vi "Configure.vi"(8 "error in (no error)":errorcluster, 10 "I2C User Configuration":T1, 11 "I2C Ref In":T3={"myRIO Reference"={"myRIO Model"=enum."Unknown", "myRIO Hardware Reference"={"Generic FPGA Reference"=refnum, "Allow multiple opens"=FALSE}}, "I2C Channels Enum"=enum."Not Connected", "I2C Configuration"={"I2C Transfer Rate"=enum."Fast mode (400 kbps)"}}) -> (0 "error out":errorcluster, 3 "I2C Ref Out":T3={"myRIO Reference"={"myRIO Model"=enum."Unknown", "myRIO Hardware Reference"={"Generic FPGA Reference"=refnum, "Allow multiple opens"=FALSE}}, "I2C Channels Enum"=enum."Not Connected", "I2C Configuration"={"I2C Transfer Rate"=enum."Fast mode (400 kbps)"}})   [LabVIEW 2021, in "I2C.lvlib"]
doc: "Configures the transfer rate of an Inter-Integrated Circuit (I2C) channel based on the input I2C reference."
uses:
  <vilib>/myRIO/Instrument Drivers/Onboard IO/I2C/I2C.lvlib
  <vilib>/myRIO/Instrument Drivers/Onboard IO/I2C/typedefs/I2C Reference.ctl
  <vilib>/myRIO/Common/Instrument Driver Framework/Utilities/typedefs/myRIO Generic Hardware Reference.ctl
  <vilib>/myRIO/Common/Instrument Driver Framework/Utilities/typedefs/Hardware Version Enum.ctl
  <vilib>/myRIO/Common/Instrument Driver Framework/Utilities/typedefs/myRIO v1.0 Reference.ctl
  <vilib>/myRIO/Common/Instrument Driver Framework/Utilities/typedefs/Generic FPGA Reference.ctl
  <vilib>/myRIO/Common/Instrument Driver Framework/myRIO v1.0/I2C/typedefs/I2C Channels Enum.ctl
  <vilib>/myRIO/Instrument Drivers/Onboard IO/I2C/typedefs/I2C Configuration.ctl
  <vilib>/myRIO/Instrument Drivers/Onboard IO/I2C/typedefs/I2C Transfer Rate.ctl
  <vilib>/myRIO/Instrument Drivers/Onboard IO/I2C/typedefs/I2C User Configuration.ctl
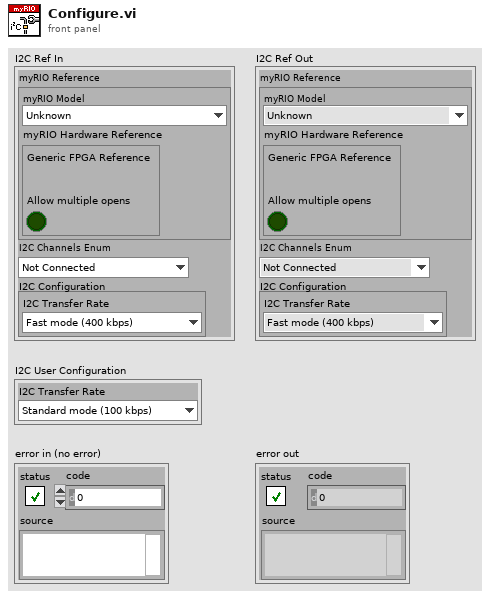
[diagram p1: front panel]
types:
  T1 = typedef "I2C.lvlib/I2C User Configuration.ctl" = cluster{"I2C Transfer Rate":T2}
  T2 = typedef "I2C.lvlib/I2C Transfer Rate.ctl" = enum16{"Standard mode (100 kbps)", "Fast mode (400 kbps)"}
  T3 = typedef "I2C.lvlib/I2C Reference.ctl" = cluster{"myRIO Reference":T4, "I2C Channels Enum":T8, "I2C Configuration":T9}
  T4 = typedef "myRIO Generic Hardware Reference.ctl" = cluster{"myRIO Model":T5, "myRIO Hardware Reference":T6}
  T5 = typedef "Hardware Version Enum.ctl" = enum16{"Unknown", "myRIO-1900", "myRIO-1950", "roboRIO", "NI ELVIS RIO CM", "ELVIS III"}
  T6 = typedef "myRIO v1.0 Reference.ctl" = cluster{"Generic FPGA Reference":T7, "Allow multiple opens":bool}
  T7 = typedef "Generic FPGA Reference.ctl" = refnum<k20>
  T8 = typedef "I2C Channels Enum.ctl" = enum16{"Not Connected", "A/I2C", "B/I2C", "I2C/I2C"}
  T9 = typedef "I2C.lvlib/I2C Configuration.ctl" = cluster{"I2C Transfer Rate":T2}
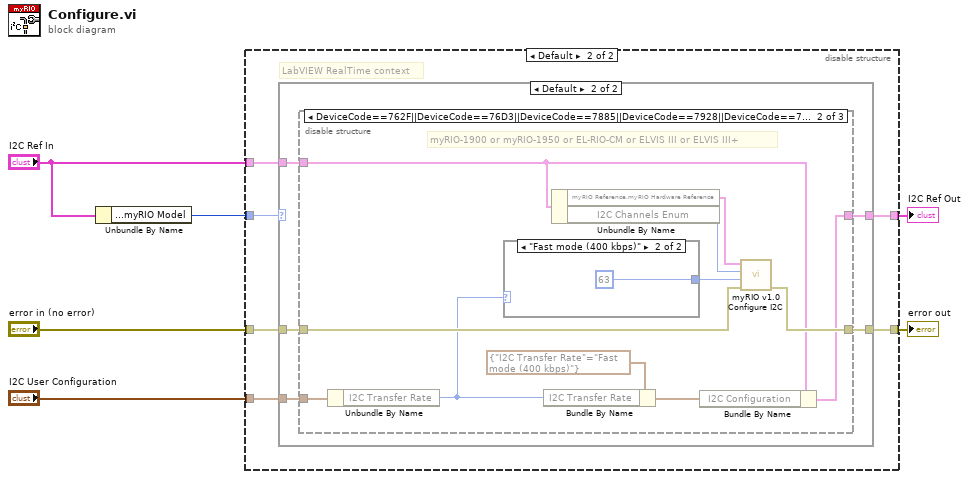
[diagram p0: block diagram]
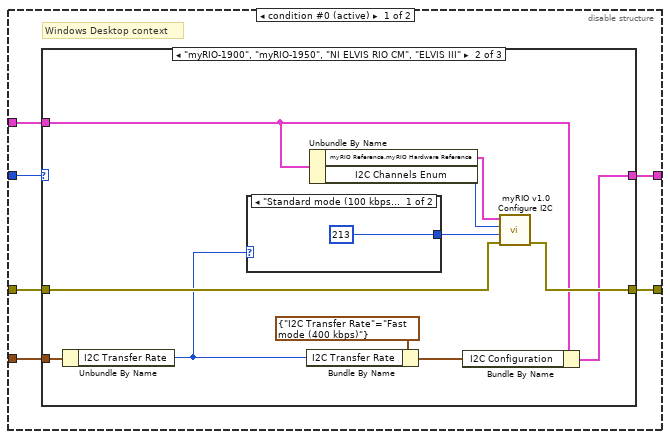
[diagram p2: hidden frame]
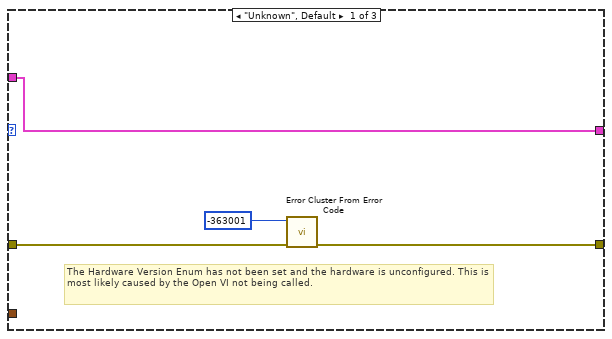
[diagram p3: hidden frame]
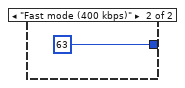
[diagram p4: hidden frame]
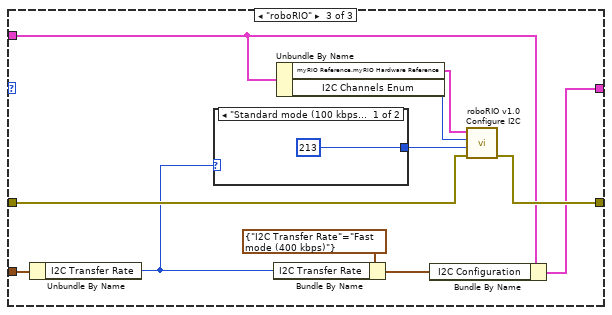
[diagram p5: hidden frame]
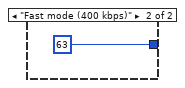
[diagram p6: hidden frame]
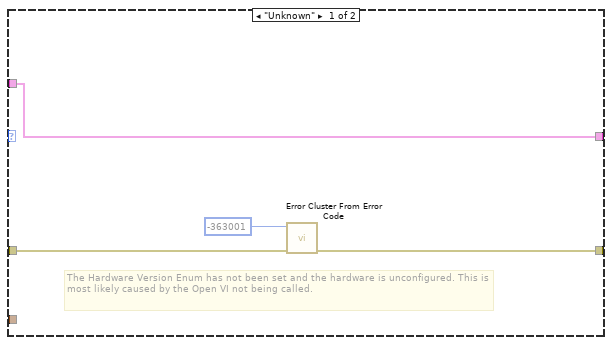
[diagram p7: hidden frame]
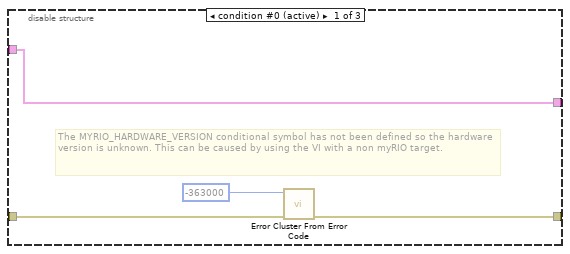
[diagram p8: hidden frame]
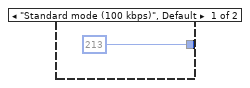
[diagram p9: hidden frame]
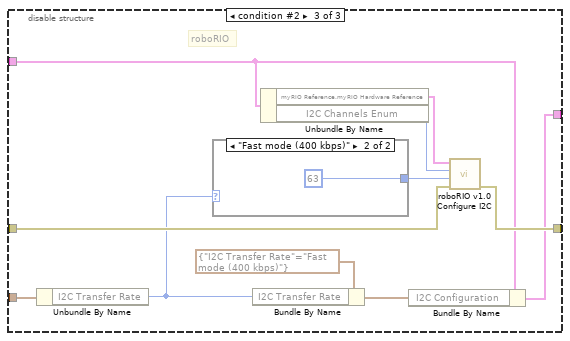
[diagram p10: hidden frame]
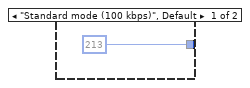
[diagram p11: hidden frame]
diagram:
  n1 = Unbundle By Name("I2C Ref In") -> ("myRIO Reference.myRIO Model"=w1:T5)
  n2 = disable-structure shown="Default" {
    disable-tunnel: [w12 w48] -> w6
    disable-tunnel: [w11 w47] -> w5
    disable-tunnel: "I2C User Configuration" -> [w10 w46]
    disable-tunnel: "I2C Ref In" -> [w9 w45]
    disable-tunnel: "error in (no error)" -> [w8 w44]
    disable-tunnel: w1 -> [w7 w43]
    frame condition #0 (active) {
      # "Windows Desktop context"
      n3 = case shown="\"myRIO-1900\", \"myRIO-1950\", \"NI ELVIS RIO CM\", \"ELVIS III\"" w7 {
        tunnel: [w15 w27 w40] -> w12
        tunnel: [w13 w26 w39] -> w11
        tunnel: w9 -> [w13 w21 w34]
        tunnel: w8 -> [w14 w25 w38]
        tunnel: w10 -> [_ w22 w35]
        frame "Unknown", Default {
          # "The Hardware Version Enum has not been set and the hardware is unconfigured. This is most likely caused by the Open VI not being called."
          n4 = call <vilib>:"Error Cluster From Error Code.vi"("error in (no error)"=w14, "error code (0)"=-363001) -> ("error out"=w15:errorcluster)  [unwired: 7 in]
        }
        frame "myRIO-1900", "myRIO-1950", "NI ELVIS RIO CM", "ELVIS III" {
          n5 = Unbundle By Name(w22) -> ("I2C Transfer Rate"=w18:T2)
          n6 = case shown="\"Standard mode (100 kbps)\", Default" w18 {
            tunnel: [u8 213 ("I2C Counter Value") u8 63 ("I2C Counter Value")] -> w17
            frame "Standard mode (100 kbps)", Default {
            }
            frame "Fast mode (400 kbps)" {
            }
          }
          n7 = Bundle By Name(cluster=T9 {"I2C Transfer Rate"=enum."Fast mode (400 kbps)"} ("I2C Configuration"), "I2C Transfer Rate"=w18) -> (w19:T9)
          n8 = Unbundle By Name(w21) -> ("myRIO Reference.myRIO Hardware Reference"=w23:T6, "I2C Channels Enum"=w24:T8)
          n9 = Bundle By Name(cluster=w21, "I2C Configuration"=w19) -> (w26:T3)
          n10 = call <vilib>:"myRIO v1.0 Configure I2C.vi"("error in (no error)"=w25, "I2C Counter Value"=w17, "Channel"=w24, "myRIO Ref In"=w23) -> ("error out"=w27:errorcluster)  [unwired: 6 in, 1 out]
        }
        frame "roboRIO" {
          n11 = Unbundle By Name(w35) -> ("I2C Transfer Rate"=w31:T2)
          n12 = case shown="\"Standard mode (100 kbps)\", Default" w31 {
            tunnel: [u8 213 ("I2C Counter Value") u8 63 ("I2C Counter Value")] -> w30
            frame "Standard mode (100 kbps)", Default {
            }
            frame "Fast mode (400 kbps)" {
            }
          }
          n13 = Bundle By Name(cluster=T9 {"I2C Transfer Rate"=enum."Fast mode (400 kbps)"} ("I2C Configuration"), "I2C Transfer Rate"=w31) -> (w32:T9)
          n14 = Unbundle By Name(w34) -> ("myRIO Reference.myRIO Hardware Reference"=w36:T6, "I2C Channels Enum"=w37:T8)
          n15 = Bundle By Name(cluster=w34, "I2C Configuration"=w32) -> (w39:T3)
          n16 = call <vilib>:"roboRIO v1.0 Configure I2C.vi"("error in (no error)"=w38, "I2C Counter Value"=w30, "Channel"=w37, "myRIO Ref In"=w36) -> ("error out"=w40:errorcluster)  [unwired: 6 in, 1 out]
        }
      }
    }
    frame condition #1 {
      # "LabVIEW RealTime context"
      n17 = case shown="Default" w43 {
        tunnel: [w51 w57] -> w48
        tunnel: [w49 w56] -> w47
        tunnel: w45 -> [w49 w53]
        tunnel: w44 -> [w50 w55]
        tunnel: w46 -> [_ w54]
        frame "Unknown" {
          # "The Hardware Version Enum has not been set and the hardware is unconfigured. This is most likely caused by the Open VI not being called."
          n18 = call <vilib>:"Error Cluster From Error Code.vi"("error in (no error)"=w50, "error code (0)"=-363001) -> ("error out"=w51:errorcluster)  [unwired: 7 in]
        }
        frame Default {
          n19 = disable-structure shown="DeviceCode==762F||DeviceCode==76D3||DeviceCode==7885||DeviceCode==7928||DeviceCode==793C" {
            disable-tunnel: [w60 w72 w85] -> w57
            disable-tunnel: [w58 w71 w84] -> w56
            disable-tunnel: w55 -> [w59 w70 w83]
            disable-tunnel: w54 -> [_ w67 w80]
            disable-tunnel: w53 -> [w58 w66 w79]
            frame condition #0 (active) {
              # "The MYRIO_HARDWARE_VERSION conditional symbol has not been defined so the hardware version is unknown. This can be caused by using the VI with a non myRIO target."
              n20 = call <vilib>:"Error Cluster From Error Code.vi"("error in (no error)"=w59, "error code (0)"=-363000) -> ("error out"=w60:errorcluster)  [unwired: 7 in]
            }
            frame condition #1 {
              # "myRIO-1900 or myRIO-1950 or EL-RIO-CM or ELVIS III or ELVIS III+"
              n21 = Unbundle By Name(w67) -> ("I2C Transfer Rate"=w63:T2)
              n22 = case shown="\"Fast mode (400 kbps)\"" w63 {
                tunnel: [u8 213 ("I2C Counter Value") u8 63 ("I2C Counter Value")] -> w62
                frame "Standard mode (100 kbps)", Default {
                }
                frame "Fast mode (400 kbps)" {
                }
              }
              n23 = Bundle By Name(cluster=T9 {"I2C Transfer Rate"=enum."Fast mode (400 kbps)"} ("I2C Configuration"), "I2C Transfer Rate"=w63) -> (w64:T9)
              n24 = Unbundle By Name(w66) -> ("myRIO Reference.myRIO Hardware Reference"=w68:T6, "I2C Channels Enum"=w69:T8)
              n25 = Bundle By Name(cluster=w66, "I2C Configuration"=w64) -> (w71:T3)
              n26 = call <vilib>:"myRIO v1.0 Configure I2C.vi"("error in (no error)"=w70, "I2C Counter Value"=w62, "Channel"=w69, "myRIO Ref In"=w68) -> ("error out"=w72:errorcluster)  [unwired: 6 in, 1 out]
            }
            frame condition #2 {
              # "roboRIO"
              n27 = Unbundle By Name(w80) -> ("I2C Transfer Rate"=w76:T2)
              n28 = case shown="\"Fast mode (400 kbps)\"" w76 {
                tunnel: [u8 213 ("I2C Counter Value") u8 63 ("I2C Counter Value")] -> w75
                frame "Standard mode (100 kbps)", Default {
                }
                frame "Fast mode (400 kbps)" {
                }
              }
              n29 = Bundle By Name(cluster=T9 {"I2C Transfer Rate"=enum."Fast mode (400 kbps)"} ("I2C Configuration"), "I2C Transfer Rate"=w76) -> (w77:T9)
              n30 = Unbundle By Name(w79) -> ("myRIO Reference.myRIO Hardware Reference"=w81:T6, "I2C Channels Enum"=w82:T8)
              n31 = Bundle By Name(cluster=w79, "I2C Configuration"=w77) -> (w84:T3)
              n32 = call <vilib>:"roboRIO v1.0 Configure I2C.vi"("error in (no error)"=w83, "I2C Counter Value"=w75, "Channel"=w82, "myRIO Ref In"=w81) -> ("error out"=w85:errorcluster)  [unwired: 6 in, 1 out]
            }
          }
        }
      }
    }
  }
  "I2C Ref Out" <- w5
  "error out" <- w6
